vi "P8_truncador.vi"() -> ()   [LabVIEW 2020]
uses:
  <vilib>/vision/NI_Vision_Development_Module.lvlib
panel:
  out "DFT Truncada":T1(plugin-control)
  in  "stop":bool
  in  "Truncamineto %":dbl(knob) scale=0.0..100.0
  out "Imagen con DFT truncada":T1(plugin-control)
  out "DFT":T1(plugin-control)
  out "Image":T1(plugin-control)
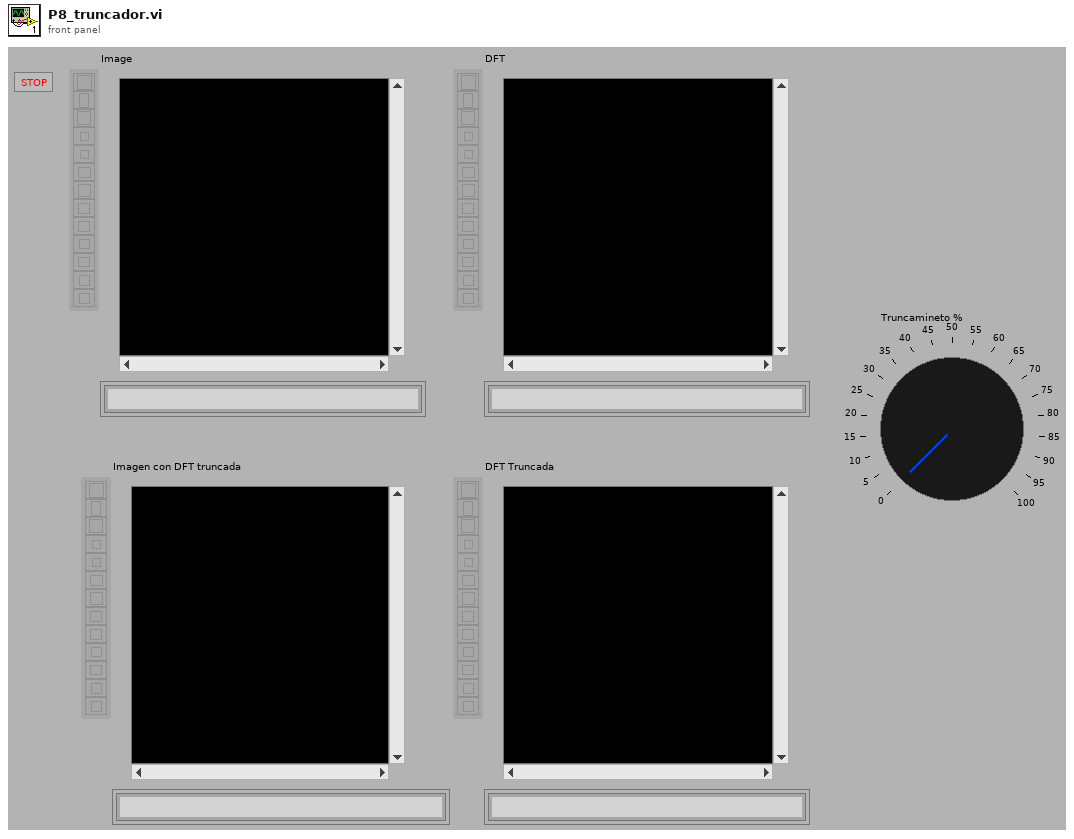
[diagram p1: front panel]
types:
  T1 = typedef "IMAQ Image.ctl" = refnum<image>
  T2 = typedef "Image Type" = u32
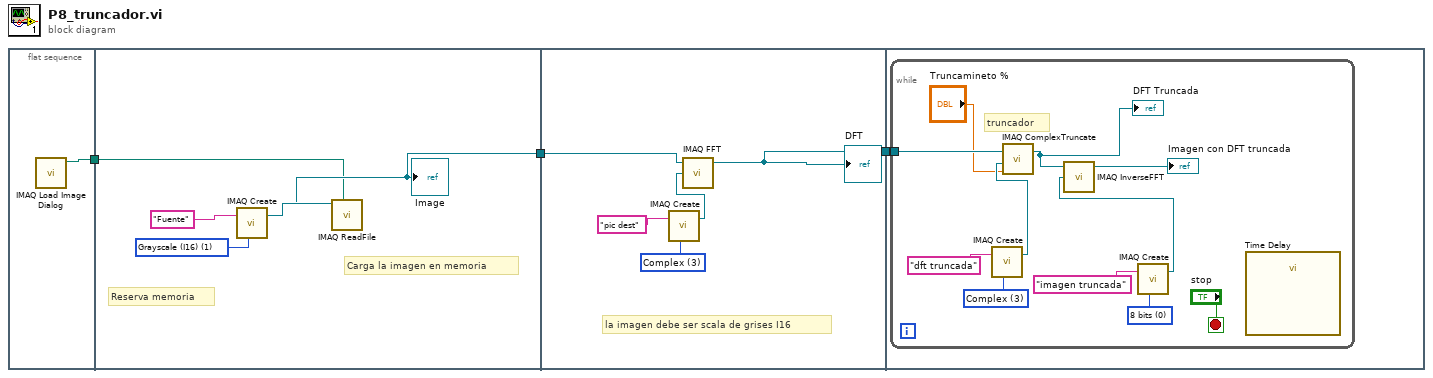
[diagram p0: block diagram]
diagram:
  n1 = flat-sequence {
    tunnel: [w4] -> w3
    tunnel: [w6] -> w2
    tunnel: w3 -> [w5]
    tunnel: w2 -> [w11]
    tunnel: [w10] -> w1
    tunnel: w1 -> [w15]
    frame #0 {
      n2 = call "IMAQ Load Image Dialog"() -> ("Path"=w4:path)  [unwired: 7 in, 4 out]
    }
    frame #1 {
      w8 = T2 1 items=["Grayscale (U8)", "Grayscale (I16)", "Grayscale (SGL)", "Complex (CSG)", "RGB (U32)", "HSL (U32)", "RGB (U64)", "Grayscale (U16)"] ("Image Type")
      # "Carga la imagen en memoria"
      # "Reserva memoria"
      n3 = call "IMAQ Create"("Image Name"="Fuente", "Image Type"=w8) -> ("New Image"=w9:T1)  [unwired: 2 in, 2 out]
      n4 = call "IMAQ ReadFile"("File Path"=w5, "Image"=w9) -> ("Image Out"=w6:T1)  [unwired: 3 in, 6 out]
      "Image" <- w6
    }
    frame #2 {
      w13 = u32 3 items=["8 bits", "16 bits", "Float", "Complex", "RGB", "HSL"] ("Image Type")
      # "la imagen debe ser scala de grises I16"
      n5 = call "IMAQ Create"("Image Name"="pic dest", "Image Type"=w13) -> ("New Image"=w14:T1)  [unwired: 2 in, 2 out]
      n6 = call "IMAQ FFT"("Image Dst"=w14, "Image Src"=w11) -> ("Image Dst Out"=w10:T1)  [unwired: 1 in, 2 out]
      "DFT" <- w10
    }
    frame #3 {
      n7 = while {
        tunnel: w15 -> [w19]
        stop <- "stop" stop-if-true
        w23 = u32 0 items=["8 bits", "16 bits", "Float", "Complex", "RGB", "HSL"] ("Image Type")
        w25 = u32 3 items=["8 bits", "16 bits", "Float", "Complex", "RGB", "HSL"] ("Image Type")
        # "truncador"
        n8 = call "IMAQ Create"("Image Name"="dft truncada", "Image Type"=w25) -> ("New Image"=w24:T1)  [unwired: 2 in, 2 out]
        n9 = call "IMAQ ComplexTruncate"("Image Dst"=w24, "Truncation Frequency %"="Truncamineto %", "Image Src"=w19) -> ("Image Dst Out"=w16:T1)  [unwired: 2 in, 3 out]
        "DFT Truncada" <- w16
        n10 = call "IMAQ Create"("Image Name"="imagen truncada", "Image Type"=w23) -> ("New Image"=w21:T1)  [unwired: 2 in, 2 out]
        n11 = call "IMAQ InverseFFT"("Image Dst"=w21, "Image Src"=w16) -> ("Image Dst Out"=→"Imagen con DFT truncada":T1)  [unwired: 1 in, 2 out]
        n12 = call "Time Delay"() -> ()  [unwired: 2 in, 10 out]
      }
    }
  }
